vi "SonarBrake.vi"() -> ()   [LabVIEW 2018]
uses:
  <vilib>/Platform/TimedLoop/XDataNode/timing_clust.ctl
  <vilib>/Platform/TimedLoop/XDataNode/nitl_modes.ctl
  <vilib>/Platform/TimedLoop/XDataNode/wakeup.ctl
  <vilib>/addons/control/pid/pid.llb/PID (DBL).vi
  <vilib>/platform/TimedLoop/XDataNode/XDataNode.xnode
  <vilib>/Platform/TimedLoop/XDataNode/XDNodeRunTimeDep.lvlib
  <vilib>/addons/control/pid/NI_PID_pid.lvlib
panel:
  in  "Tab Control":enum32{"Sonar"}(tab)
  in  "Tol (sec)":dbl=0.25 format="%#_13g"
  in  "Tol (in)":dbl=1.1
  out "Arrived":bool
  out "Error":dbl=3.6889665140000005
  in  "Rate Thresh":dbl=100.0 format="%#_13g"
  out "OOR":bool
  out "Mode":bool=TRUE
  in  "hi limit":dbl=200.0
  out "Strobe":bool
  in  "setpoint":dbl=20.0 format="%.2f"
  out "Sonar PID":cluster{"setpoint":dbl, "Filtered":dbl, i16}(graph)={"setpoint"=20.0, "Filtered"=25.026852906000002, 0}
  in  "Use Enc?":bool
  out "Sonar error":dbl=-5.026852906000002
  in  "clamp":cluster{"output high":dbl, "output low":dbl}={"output high"=0.65, "output low"=-0.65} {"output low" format="%.2f"; "output high" format="%.2f"}
  in  "PID gains":T1={"proportional gain (Kc)"=0.01, "integral time (Ti, min)"=0.0, "derivative time (Td, min)"=0.003} {"derivative time (Td, min)" format="%.5f"; "integral time (Ti, min)" format="%.3f"; "proportional gain (Kc)" format="%.3f"}
  out "Sonar Left":cluster{"Filtered":dbl, dbl}(graph)={"Filtered"=16.311033486, 16.311033486}
  out "Sonar Late?":bool
  in  "Period":i64=5
  in  "Reset Enc":bool
  out "Enc":dbl=-175.22221640625
  # "Real Time Data Repair"
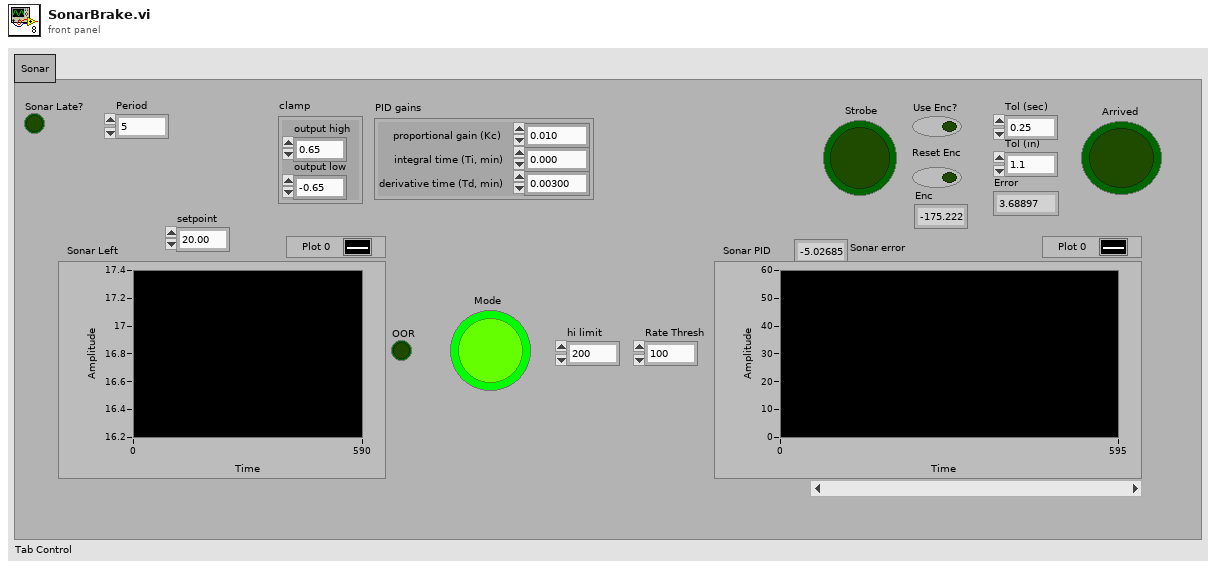
[diagram p1: front panel]
types:
  T1 = cluster{"proportional gain (Kc)":dbl, "integral time (Ti, min)":dbl, "derivative time (Td, min)":dbl}
  T2 = typedef "WPI_AnalogChannelDevRef.ctl" = cluster{"DevStatus":errorcluster, "Analog Channel":T3}
  T3 = typedef "FPGA_AIChannel.ctl" = enum8{"AI 0", "AI 1", "AI 2", "AI 3", "AI MXP 0", "AI MXP 1", "AI MXP 2", "AI MXP 3", "Invalid"}
  T4 = typedef "XDNodeRunTimeDep.lvlib/timing_clust.ctl" = cluster{"Expected End [f-1]":u64, "Actual End [f-1]":u64, "Finished Late? [f-1]":bool, "Expected End [i-1]":u64, "Actual End [i-1]":u64, "Finished Late? [i-1]":bool, "Expected Start [i]":u64, "Actual Start [i]":u64, "Expected Start [f]":u64, "Actual Start [f]":u64, "Source Name":string, "Structure Name":string, "Period":i64, "Deadline":i64, "Offset":i64, "Start":i64, "Priority":i32, "Timeout":i32, "Mode":T5, "Wakeup Reason":T6, "Error":errorcluster, "Source Type":string, "Secondary Source Type":string, "Global End Time":u64, "Global Start Time":u64, "Frame Duration":u64, "Iteration Duration":u64, "Assigned CPU":i32, "I/O Scan Engine Mode":u32}
  T5 = typedef "XDNodeRunTimeDep.lvlib/nitl_modes.ctl" = enum32{"No Change", "Process missed periods, maintain original phase", "Discard missed periods, maintain original phase", "Process missed periods, ignore original phase", "Discard missed periods, ignore original phase"}
  T6 = typedef "XDNodeRunTimeDep.lvlib/wakeup.ctl" = enum32{"Normal", "Aborted", "Asynchronous wakeup", "Timing source error", "Timed loop error", "Timeout"}
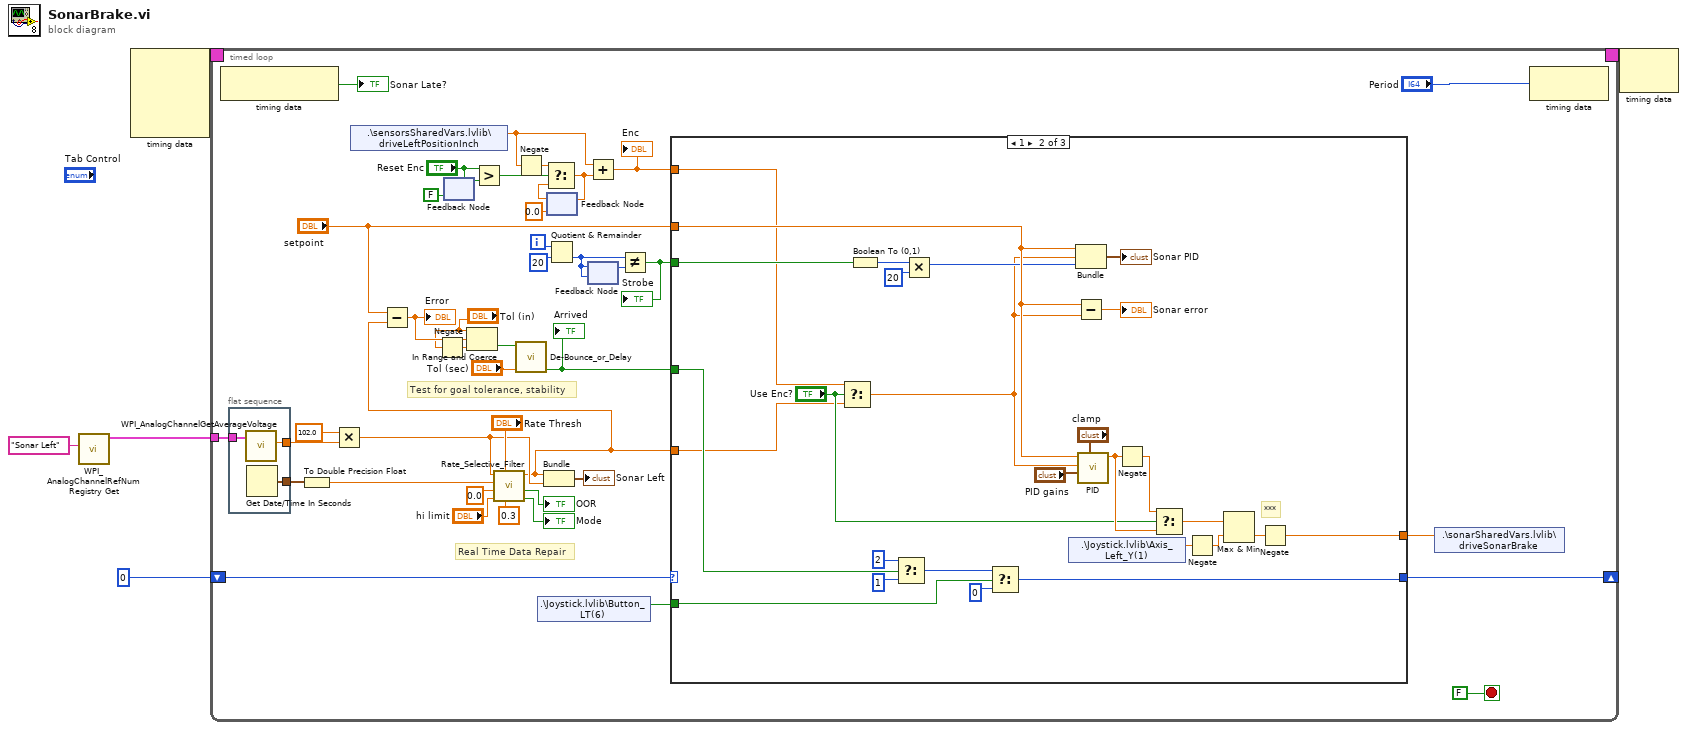
[diagram p0: block diagram]
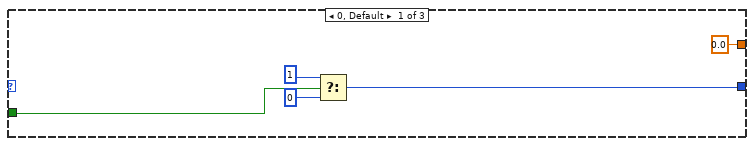
[diagram p2: hidden frame]
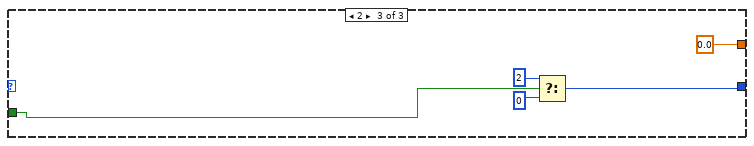
[diagram p3: hidden frame]
diagram:
  n1 = call <vilib>:"WPI_AnalogChannelRefNum Registry Get.vi"("refnum name"="Sonar Left") -> ("AIDeviceRef"=w2:T2)  [unwired: 9 in, 1 out]
  n2 = node-c288() -> (w5:T4)  [unwired: 4 in]
  n3 = timed-loop {
    timing: w5 -> [_]
    timing-out: [_] -> w4
    tunnel: w2 -> [w46]
    shift-right: [w44] -> _
    shift-left: 0 -> [w43]
    i -> [w39]
    stop <- FALSE stop-if-true
    # "Real Time Data Repair"
    # "Test for goal tolerance, stability"
    n4 = node-c288() -> (→"Sonar Late?":bool)  [unwired: 1 in]
    n5 = flat-sequence {
      tunnel: [w51] -> w29
      tunnel: w46 -> [w50]
      tunnel: [w49] -> w36
      frame #0 {
        n6 = call <vilib>:"WPI_AnalogChannelGetAverageVoltage.vi"("AIDeviceRef"=w50) -> ("Voltage"=w51:dbl)  [unwired: 8 in, 2 out]
        n7 = Get Date/Time In Seconds() -> (seconds since 1Jan1904=w49:timestamp)
      }
    }
    n8 = To Double Precision Float(number=w36) -> (double precision float=w35:dbl)
    n9 = Multiply(x=102.0, y=w29) -> (x*y=w20:dbl)
    n10 = shared-variable ".\\sensorsSharedVars.lvlib\\driveLeftPositionInch"() -> (w9:dbl)  [unwired: 1 in, 1 out]
    n11 = Negate(x="Tol (in)") -> (-x=w27:dbl)
    n12 = feedback #1(FALSE ("Reset Enc")) -> (w14:bool)
    n13 = feedback-in #1("Reset Enc") -> ()
    n14 = Greater?(x="Reset Enc", y=w14) -> (0:w16:bool)
    n15 = call <userlib>:"Rate_Selective_Filter.vi"("Hyster"=0.3, "Rate Thresh"="Rate Thresh", "hi limit"="hi limit", "lo limit"=0.0, "Time"=w35, "Distance"=w20) -> ("Mode"=→"Mode":bool, "OOR"=→"OOR":bool, "Filtered"=w7:dbl)  [unwired: 1 in]
    n16 = Subtract(x="setpoint", y=w7) -> (x-y=w28:dbl)
    "Error" <- w28
    n17 = In Range and Coerce(upper limit="Tol (in)", x=w28, lower limit=w27) -> (In Range?=w25:bool)  [unwired: 1 out]
    n18 = Negate(x=w9) -> (-x=w17:dbl)
    n19 = call <userlib>:"De-Bounce_or_Delay.vi"("Eval Period (sec)"="Tol (sec)", "Signal Input"=w25) -> ("Stable"=w22:bool)  [unwired: 9 in]
    "Arrived" <- w22
    n20 = shared-variable ".\\Joystick.lvlib\\Button_LT(6)"() -> (w18:bool)  [unwired: 1 in, 1 out]
    n21 = Bundle("Filtered"=w7, w20) -> (→"Sonar Left":cluster{"Filtered":dbl, dbl})  [unwired: 1 in]
    n22 = feedback #2(0.0) -> (w11:dbl)
    n23 = Select(t=w17, s=w16, f=w11) -> (s? t:f=w8:dbl)
    n24 = feedback-in #2(w8) -> ()
    n25 = Quotient & Remainder(x=w39, y=20) -> (floor(x/y)=w42:i32)  [unwired: 1 out]
    n26 = Add(x=w9, y=w8) -> (x+y=w10:dbl)
    "Enc" <- w10
    n27 = feedback #3(w42) -> (w41:i32)
    n28 = feedback-in #3(w42) -> ()
    n29 = Not Equal?(x=w42, y=w41) -> (x != y?=w21:bool)
    "Strobe" <- w21
    n30 = case shown="1" w43 {
      tunnel: [w55 w81 w86] -> w44
      tunnel: w18 -> [w53 w80 w85]
      tunnel: "setpoint" -> [_ w66 _]
      tunnel: w10 -> [_ w62 _]
      tunnel: w21 -> [_ w75 _]
      tunnel: w7 -> [_ w67 _]
      tunnel: w22 -> [_ w71 _]
      tunnel: [0.0 ("Left Drive") w57 0.0 ("Left Drive")] -> w6
      frame 0, Default {
        n31 = Select(t=1, s=w53, f=0) -> (s? t:f=w55:i32)
      }
      frame 1 {
        # "***"
        n32 = Select(t=w62, s="Use Enc?", f=w67) -> (s? t:f=w63:dbl)
        n33 = Boolean To (0,1)(Boolean=w75) -> (0, 1=w76:i16)
        n34 = Select(t=2, s=w71, f=1) -> (s? t:f=w68:i32)
        n35 = Multiply(x=w76, y=i16 20) -> (x*y=w64:i16)
        n36 = Select(t=w68, s=w80, f=0) -> (s? t:f=w81:i32)
        n37 = shared-variable ".\\Joystick.lvlib\\Axis_Left_Y(1)"() -> (w61:dbl)  [unwired: 1 in, 1 out]
        n38 = Bundle("setpoint"=w66, "Filtered"=w63, w64) -> (→"Sonar PID":cluster{"setpoint":dbl, "Filtered":dbl, i16})  [unwired: 1 in]
        n39 = Subtract(x=w66, y=w63) -> (x-y=→"Sonar error":dbl)
        n40 = call-poly <vilib>:"PID.vi"("output range"="clamp", "PID gains"="PID gains", "process variable"=w63, "setpoint"=w66) -> ("output"=w79:dbl)  [unwired: 6 in, 1 out]
        n41 = Negate(x=w79) -> (-x=w78:dbl)
        n42 = Select(t=w78, s="Use Enc?", f=w79) -> (s? t:f=w58:dbl)
        n43 = Negate(x=w61) -> (-x=w60:dbl)
        n44 = Max & Min(x=w58, y=w60) -> (min(x,y)=w59:dbl)  [unwired: 1 out]
        n45 = Negate(x=w59) -> (-x=w57:dbl)
      }
      frame 2 {
        n46 = Select(t=2, s=w85, f=0) -> (s? t:f=w86:i32)
      }
    }
    n47 = shared-variable ".\\sonarSharedVars.lvlib\\driveSonarBrake"(w6) -> ()  [unwired: 1 in, 1 out]
    n48 = node-c288("Period") -> ()  [unwired: 1 out]
  }
  n49 = node-c288(w4) -> ()  [unwired: 1 out]
